vi "Untitled 2.vi"(9 "Index  per standard":i32, 10 "Select Standard":T5={"Tx_ 802.11a/g OFDM"=TRUE, "Tx_ 802.11b DSSS/CCK"=TRUE, "Tx_ 802.11n OFDM "=TRUE, "Tx_ 802.11ac OFDM "=FALSE}, 11 "stard":i32) -> (3 "Command Sent":string)   [LabVIEW 2011]
uses:
  niWLAN/WLAN -  niWLAN - INC - Select Measurement.ctl
  TV/RW/Includes/WLAN - TV - RW - INC - TV_DataType_Cluster.ctl
  TV/RW/Includes/WLAN - TV - RW - INC - Tx_Measurement_Cluster.ctl
  TV/RW/Includes/WLAN - TV - RW - INC - TV_OFDM Demod.ctl
  TV/RW/Includes/WLAN - TV - RW - INC - TV_DSSS Demod.ctl
panel:
  out "TV Test Seq":path[](array[path])
  out "TV":T1 {"Standard" items=["80211A/G/J/P OFDM", "80211B/G DSSS", "80211G DSSSOFDM", "80211N MIMOOFDM", "80211AC MIMOOFDM"]; "OFDM Data Rate (Mbps)" items=["6", "9", "12", "18", "24", "36", "48", "54"]; "80211n PLCP Frame Format" items=["Mixed Format", "Greenfield Format"]; "FEC Coding Type" items=["BCC", "LDPC"]; "DSSS Data Rate (Mbps)" items=["1", "2", "5.5 CCK", "5.5 PBCC", "11 CCK", "11 PBCC", "22", "33"]}
  out "size(s)":i32
  out "WLAN Measurement Settings":T2={"OFDM Advanced Controls(11ag)"={"OFDM Auto Compute Acquisition Length Enabled"=0, "OFDM Maximum Symbols Used"=0, "OFDM Time Tracking Enabled"=0, "OFDM Channel Tracking Enabled"=0, "OFDM Amplitude Tracking Enabled"=1, "OFDM CFO Estimation Method"=0, "OFDM Phase Tracking Method"=0, "OFDM Header Detection Enabled"=0, "OFDM MAC FCS Check Enabled"=0, "#Avg"=10, "#Iterations"=10}, "DSSS Demod Parameters"={"DSSS Auto Compute Acquisition Length Enabled"=0, "DSSS Equalization Enabled"=0, "DSSS Header Detection Enabled"=0, "DSSS MAC FCS Check Enabled"=0, "DSSS Measurement Start Location"=0, "DSSS Phase Tracking Method"=0, "DSSS Maximum Chips Used"=0, "DSSS Reference Pulse Shaping Filter"=0, "DSSS Reference Pulse Shaping Filter Coefficient"=0.0, "# Avg"=1024, "# Iterations"=1024, "DSSS Power Ramp Enabled"=0}, "OFDM Advanced Controls (11n)"={"OFDM Auto Compute Acquisition Length Enabled"=0, "OFDM Maximum Symbols Used"=0, "OFDM Time Tracking Enabled"=0, "OFDM Channel Tracking Enabled"=0, "OFDM Amplitude Tracking Enabled"=1, "OFDM CFO Estimation Method"=0, "OFDM Phase Tracking Method"=0, "OFDM Header Detection Enabled"=0, "OFDM MAC FCS Check Enabled"=0, "#Avg"=10, "#Iterations"=10}, "OFDM Advanced Controls(11ac)"={"OFDM Auto Compute Acquisition Length Enabled"=0, "OFDM Maximum Symbols Used"=0, "OFDM Time Tracking Enabled"=1, "OFDM Channel Tracking Enabled"=0, "OFDM Amplitude Tracking Enabled"=0, "OFDM CFO Estimation Method"=0, "OFDM Phase Tracking Method"=0, "OFDM Header Detection Enabled"=0, "OFDM MAC FCS Check Enabled"=0, "#Avg"=10, "#Iterations"=10}} {"OFDM Advanced Controls(11ac)"."OFDM Phase Tracking Method" items=["Standard", "Instantaneous", "None", "Standard with Cubic Spline Fit"]; "OFDM Advanced Controls(11ac)"."OFDM CFO Estimation Method" items=["Preamble Only", "Preamble and Data"]; "OFDM Advanced Controls(11ac)"."OFDM Channel Tracking Enabled" items=["False", "True"]; "OFDM Advanced Controls(11ac)"."OFDM Amplitude Tracking Enabled" items=["False", "True"]; "OFDM Advanced Controls(11ac)"."OFDM Time Tracking Enabled" items=["True"=1, "False"=0]; "OFDM Advanced Controls(11ac)"."OFDM Auto Compute Acquisition Length Enabled" items=["False", "True"]; "OFDM Advanced Controls(11ac)"."OFDM MAC FCS Check Enabled" items=["False", "True"]; "OFDM Advanced Controls(11ac)"."OFDM Header Detection Enabled" items=["False", "True"]; "OFDM Advanced Controls (11n)"."OFDM Phase Tracking Method" items=["Standard", "Instantaneous", "None", "Standard with Cubic Spline Fit"]; "OFDM Advanced Controls (11n)"."OFDM CFO Estimation Method" items=["Preamble Only", "Preamble and Data"]; "OFDM Advanced Controls (11n)"."OFDM Channel Tracking Enabled" items=["False", "True"]; "OFDM Advanced Controls (11n)"."OFDM Amplitude Tracking Enabled" items=["False", "True"]; "OFDM Advanced Controls (11n)"."OFDM Time Tracking Enabled" items=["True"=1, "False"=0]; "OFDM Advanced Controls (11n)"."OFDM Auto Compute Acquisition Length Enabled" items=["False", "True"]; "OFDM Advanced Controls (11n)"."OFDM MAC FCS Check Enabled" items=["False", "True"]; "OFDM Advanced Controls (11n)"."OFDM Header Detection Enabled" items=["False", "True"]; "DSSS Demod Parameters"."DSSS Power Ramp Enabled" items=["False", "True"]; "DSSS Demod Parameters"."DSSS Auto Compute Acquisition Length Enabled" items=["False", "True"]; "DSSS Demod Parameters"."DSSS Phase Tracking Method" items=["Standard", "Instantaneous"]; "DSSS Demod Parameters"."DSSS Equalization Enabled" items=["False", "True"]; "DSSS Demod Parameters"."DSSS Reference Pulse Shaping Filter" items=["Rectangular", "Raised Cosine", "Root Raised Cosine", "Gaussian"]; "DSSS Demod Parameters"."DSSS MAC FCS Check Enabled" items=["False", "True"]; "DSSS Demod Parameters"."DSSS Header Detection Enabled" items=["False", "True"]; "OFDM Advanced Controls(11ag)"."OFDM Phase Tracking Method" items=["Standard", "Instantaneous", "None", "Standard with Cubic Spline Fit"]; "OFDM Advanced Controls(11ag)"."OFDM CFO Estimation Method" items=["Preamble Only", "Preamble and Data"]; "OFDM Advanced Controls(11ag)"."OFDM Channel Tracking Enabled" items=["False", "True"]; "OFDM Advanced Controls(11ag)"."OFDM Amplitude Tracking Enabled" items=["False", "True"]; "OFDM Advanced Controls(11ag)"."OFDM Time Tracking Enabled" items=["True"=1, "False"=0]; "OFDM Advanced Controls(11ag)"."OFDM Auto Compute Acquisition Length Enabled" items=["False", "True"]; "OFDM Advanced Controls(11ag)"."OFDM MAC FCS Check Enabled" items=["False", "True"]; "OFDM Advanced Controls(11ag)"."OFDM Header Detection Enabled" items=["False", "True"]}
  out "Tv First Element":T1 {"Standard" items=["80211A/G/J/P OFDM", "80211B/G DSSS", "80211G DSSSOFDM", "80211N MIMOOFDM", "80211AC MIMOOFDM"]; "OFDM Data Rate (Mbps)" items=["6", "9", "12", "18", "24", "36", "48", "54"]; "80211n PLCP Frame Format" items=["Mixed Format", "Greenfield Format"]; "FEC Coding Type" items=["BCC", "LDPC"]; "DSSS Data Rate (Mbps)" items=["1", "2", "5.5 CCK", "5.5 PBCC", "11 CCK", "11 PBCC", "22", "33"]}
  out "TV's":T1[](array[typedef]) {"Standard" items=["80211A/G/J/P OFDM", "80211B/G DSSS", "80211G DSSSOFDM", "80211N MIMOOFDM", "80211AC MIMOOFDM"]; "OFDM Data Rate (Mbps)" items=["6", "9", "12", "18", "24", "36", "48", "54"]; "80211n PLCP Frame Format" items=["Mixed Format", "Greenfield Format"]; "FEC Coding Type" items=["BCC", "LDPC"]; "DSSS Data Rate (Mbps)" items=["1", "2", "5.5 CCK", "5.5 PBCC", "11 CCK", "11 PBCC", "22", "33"]}
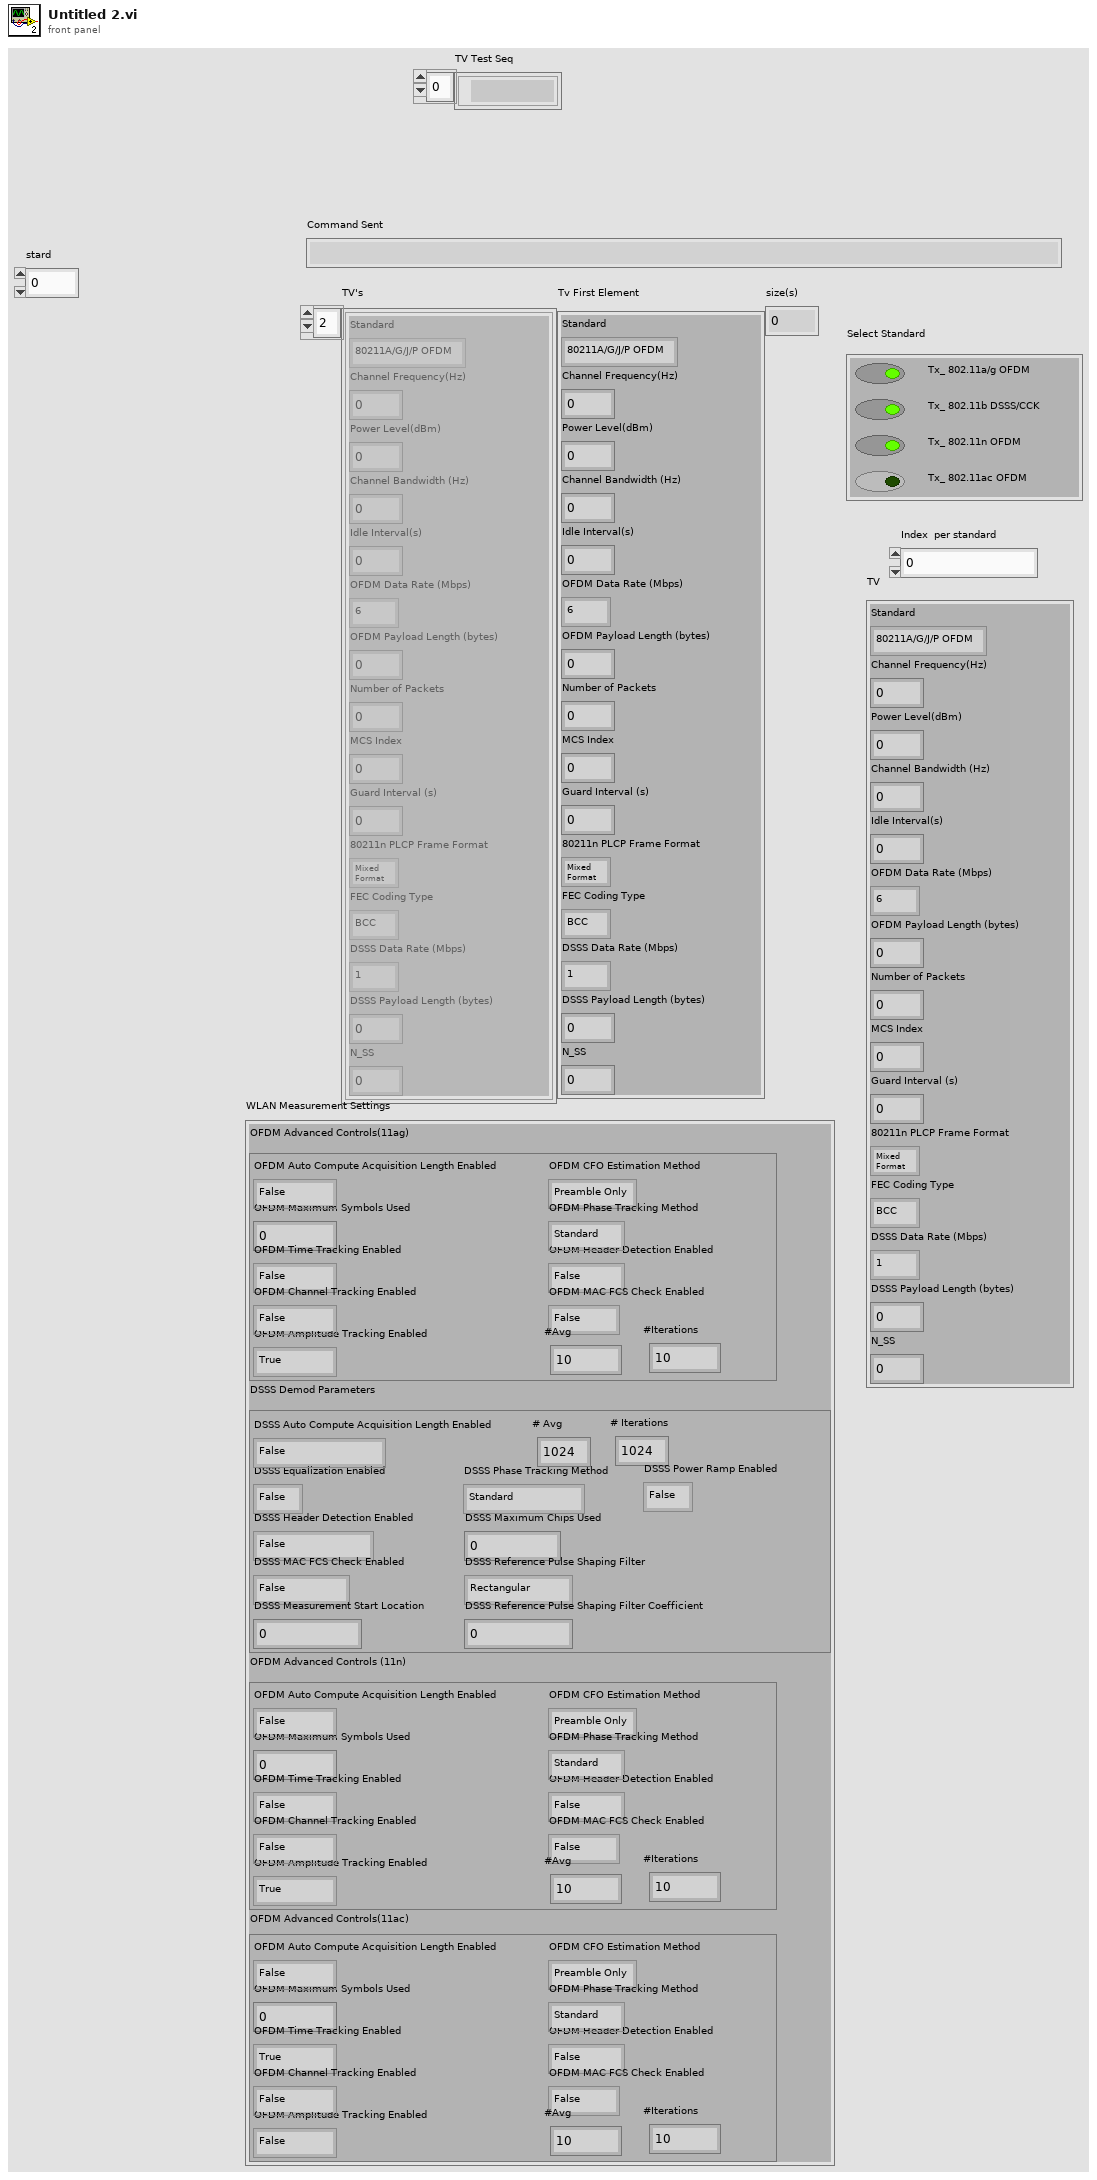
[diagram p1: front panel]
types:
  T1 = typedef "WLAN - TV - RW - INC - TV_DataType_Cluster.ctl" = cluster{"Standard":i32, "Channel Frequency(Hz)":dbl, "Power Level(dBm)":dbl, "Channel Bandwidth (Hz)":dbl, "Idle Interval(s)":dbl, "OFDM Data Rate (Mbps)":i32, "OFDM Payload Length (bytes)":i32, "Number of Packets":i32, "MCS Index":i32, "Guard Interval (s)":dbl, "80211n PLCP Frame Format":i32, "FEC Coding Type":i32, "DSSS Data Rate (Mbps)":i32, "DSSS Payload Length (bytes)":i32, "N_SS":i32}
  T2 = typedef "WLAN - TV - RW - INC - Tx_Measurement_Cluster.ctl" = cluster{"OFDM Advanced Controls(11ag)":T3, "DSSS Demod Parameters":T4, "OFDM Advanced Controls (11n)":T3, "OFDM Advanced Controls(11ac)":cluster{"OFDM Auto Compute Acquisition Length Enabled":i32, "OFDM Maximum Symbols Used":i32, "OFDM Time Tracking Enabled":i32, "OFDM Channel Tracking Enabled":i32, "OFDM Amplitude Tracking Enabled":i32, "OFDM CFO Estimation Method":i32, "OFDM Phase Tracking Method":i32, "OFDM Header Detection Enabled":i32, "OFDM MAC FCS Check Enabled":i32, "#Avg":i32, "#Iterations":i32}}
  T3 = typedef "WLAN - TV - RW - INC - TV_OFDM Demod.ctl" = cluster{"OFDM Auto Compute Acquisition Length Enabled":i32, "OFDM Maximum Symbols Used":i32, "OFDM Time Tracking Enabled":i32, "OFDM Channel Tracking Enabled":i32, "OFDM Amplitude Tracking Enabled":i32, "OFDM CFO Estimation Method":i32, "OFDM Phase Tracking Method":i32, "OFDM Header Detection Enabled":i32, "OFDM MAC FCS Check Enabled":i32, "#Avg":i32, "#Iterations":i32}
  T4 = typedef "WLAN - TV - RW - INC - TV_DSSS Demod.ctl" = cluster{"DSSS Auto Compute Acquisition Length Enabled":i32, "DSSS Equalization Enabled":i32, "DSSS Header Detection Enabled":i32, "DSSS MAC FCS Check Enabled":i32, "DSSS Measurement Start Location":i32, "DSSS Phase Tracking Method":i32, "DSSS Maximum Chips Used":i32, "DSSS Reference Pulse Shaping Filter":i32, "DSSS Reference Pulse Shaping Filter Coefficient":dbl, "# Avg":i32, "# Iterations":i32, "DSSS Power Ramp Enabled":i32}
  T5 = typedef "WLAN -  niWLAN - INC - Select Measurement.ctl" = cluster{"Tx_ 802.11a/g OFDM":bool, "Tx_ 802.11b DSSS/CCK":bool, "Tx_ 802.11n OFDM ":bool, "Tx_ 802.11ac OFDM ":bool}
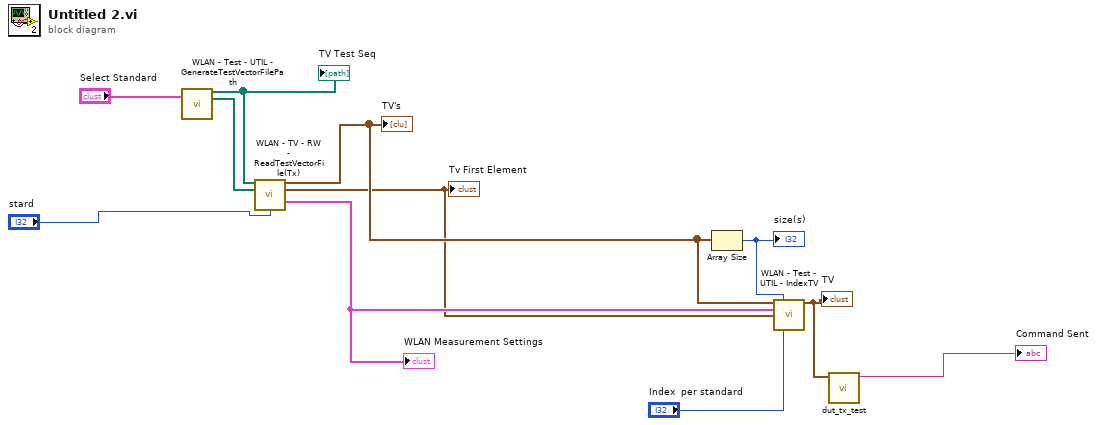
[diagram p0: block diagram]
diagram:
  n1 = call "WLAN - Test - UTIL - GenerateTestVectorFilePath.vi"("Select Measurement"="Select Standard") -> ("TV Test Seq"=w10:path[], "TV Meas Config"=w9:path[])  [unwired: 11 in, 2 out]
  "TV Test Seq" <- w10
  n2 = call "WLAN - TV - RW - ReadTestVectorFile(Tx).vi"("TX_TV_Sequence"=w10, "Measurment Settings"=w9, "Index"="stard") -> ("TV's"=w7:T1[], "Tv First Element"=w5:T1, "WLAN Measurement Settings"=w6:T2)  [unwired: 8 in, 2 out]
  "TV's" <- w7
  "Tv First Element" <- w5
  "WLAN Measurement Settings" <- w6
  n3 = Array Size(array=w7) -> (size(s)=w3:i32)
  "size(s)" <- w3
  n4 = call "WLAN - Test - UTIL - IndexTV.vi"("TV"=w7, "N"=w3, "WLAN Measurement Settings"=w6, "Tv First Element"=w5, "Index"="Index  per standard") -> ("TV"=w2:T1)  [unwired: 8 in, 2 out]
  "TV" <- w2
  n5 = call "dut_tx_test.vi"("TV Parameters(DataType)"=w2) -> ("Command Sent"=→"Command Sent":string)  [unwired: 10 in]
